vi "SetDetect(SubVI).vi"(9 "pressure":sgl, 10 "led selected":u8 format="%x", 11 "sn":string) -> (3 "output frame":string)   [LabVIEW 2012]
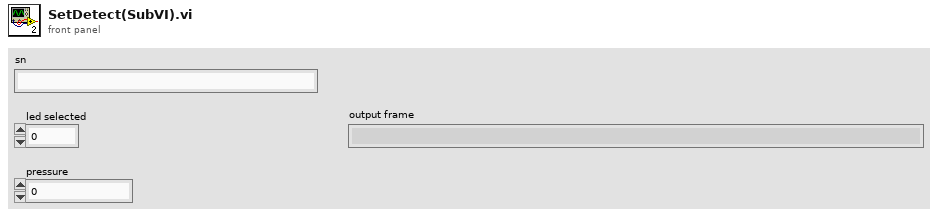
[diagram p1: front panel]
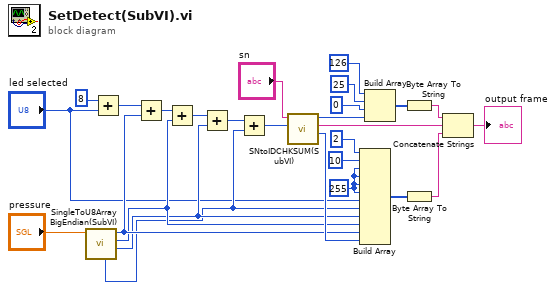
[diagram p0: block diagram]
diagram:
  w21 = u8 255
  n1 = call "SingleToU8ArrayBigEndian(SubVI).vi"("long data"="pressure") -> ("third byte"=w24:u8, "send byte"=w25:u8, "first byte"=w26:u8, "forth byte"=w23:u8)  [unwired: 7 in]
  n2 = Add(x=u8 8, y="led selected") -> (x+y=w13:u8)
  n3 = Add(x=w13, y=w26) -> (x+y=w14:u8)
  n4 = Add(x=w14, y=w25) -> (x+y=w15:u8)
  n5 = Add(x=w15, y=w24) -> (x+y=w16:u8)
  n6 = Add(x=w16, y=w23) -> (x+y=w17:u8)
  n7 = call "SNtoIDCHKSUM(SubVI).vi"("fix cheksum"=w17, "input sn"="sn") -> ("output check sum"=w27:u8, "output sn"=w7:string, "output id"=w3:u8)  [unwired: 7 in]
  n8 = Build Array(u8 2, u8 10, w21, w21, w21, w21, "led selected", w23, w24, w25, w26, w27) -> (w8:u8[])
  n9 = Build Array(u8 126, u8 25, u8 0, w3) -> (w5:u8[])
  n10 = Byte Array To String(unsigned byte array=w5) -> (string=w6:string)
  n11 = Byte Array To String(unsigned byte array=w8) -> (string=w9:string)
  n12 = Concatenate Strings(w6, w7, w9) -> (→"output frame":string)
